vi "PID unit_re.vi"(0 "dt":dbl=1.0 format="%0.2f", 4 "Kd":dbl=30.0, 5 "PID":bool, 6 "현재 온도":dbl[](array[numeric]), 7 "Ki":dbl=50.0, 8 "Kp":dbl=20.0, 9 "Target 온도":dbl=10.0) -> (3 "적정 PRF":dbl=-95.93375)   [LabVIEW 2016]
uses:
  <vilib>/Analysis/2dsp.llb/Derivative x(t).vi
  <vilib>/Analysis/NI_AALPro.lvlib
panel:
  out "Current T":dbl
  out "Integral X":dbl[](array[numeric]) format="%0.2f"
  out "x-y":dbl[](array[numeric])
  out "Sequence(i)":i32
  out "reversed array":dbl[](array[numeric])
  out "Diff":dbl
  out "Temperature chart":dbl(graph)
  out "dX/dt":dbl[](array[numeric]) format="%0.2f"
  out "array w/ subset deleted":dbl[](array[numeric])=[-30.25, -30.5, -30.75, -31.0, -31.25, -31.5, -31.75, -32.0]
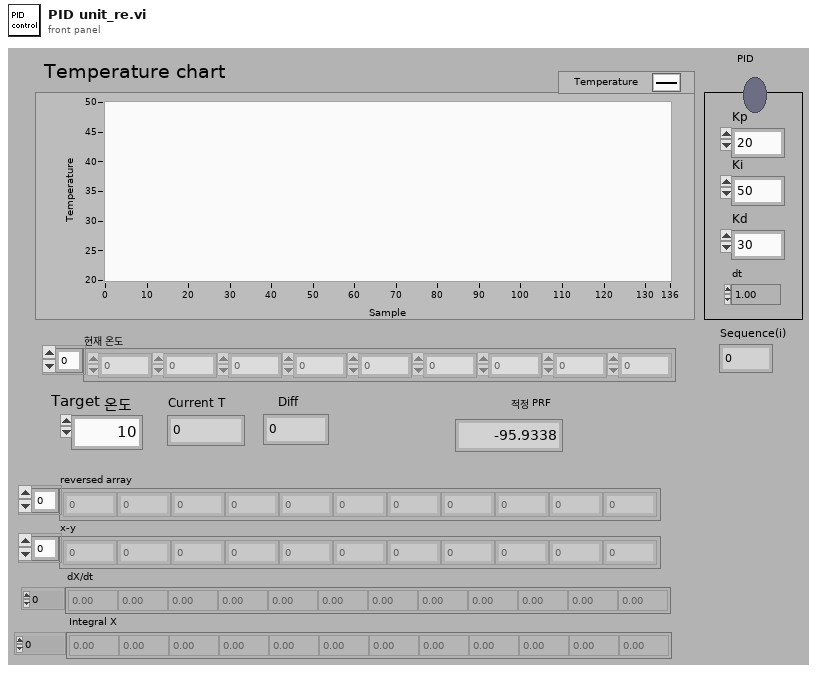
[diagram p1: front panel]
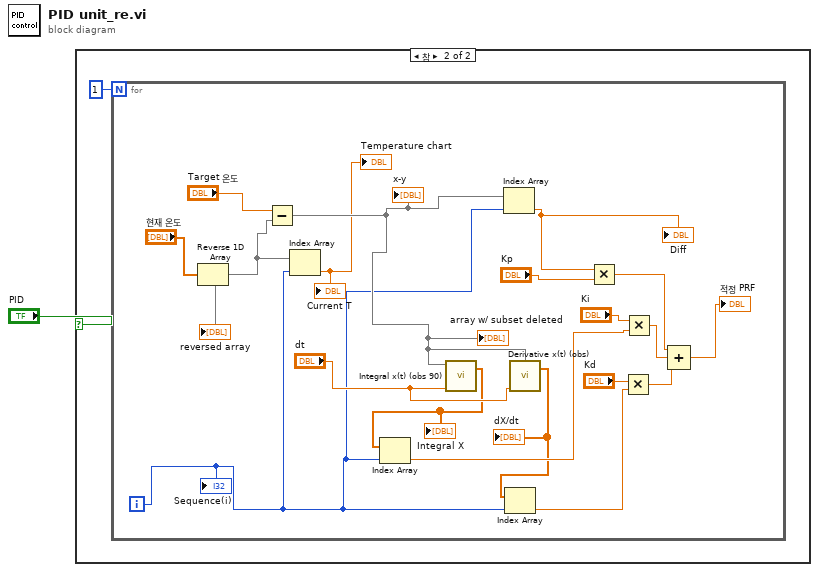
[diagram p0: block diagram]
diagram:
  n1 = case shown="참" "PID" {
    frame False {
    }
    frame True {
      n2 = for {
        N: 1 -> [_]
        i -> [w6]
        n3 = Reverse 1D Array(array="현재 온도") -> (reversed array=w4:dbl[])
        "reversed array" <- w4
        n4 = Subtract(x="Target 온도", y=w4) -> (x-y=w9:dbl[])
        "array w/ subset deleted" <- w9
        "x-y" <- w9
        n5 = Index Array(array=w4, index=w6) -> (element=→"Temperature chart" →"Current T":dbl)
        n6 = call <vilib>:"Integral x(t) (obs 90).vi"("dt"="dt", "X"=w9) -> ("Integral X"=w13:dbl[])  [unwired: 2 in, 1 out]
        "Integral X" <- w13
        n7 = Index Array(array=w13, index=w6) -> (element=w12:dbl)
        n8 = Index Array(array=w9, index=w6) -> (element=w8:dbl)
        "Diff" <- w8
        n9 = call <vilib>:"Derivative x(t) (obs).vi"("dt"="dt", "X"=w9) -> ("dX/dt"=w11:dbl[])  [unwired: 2 in, 1 out]
        "dX/dt" <- w11
        n10 = Index Array(array=w11, index=w6) -> (element=w10:dbl)
        n11 = Multiply(x=w8, y="Kp") -> (x*y=w21:dbl)
        n12 = Multiply(x="Kd", y=w10) -> (x*y=w15:dbl)
        n13 = Multiply(x="Ki", y=w12) -> (x*y=w14:dbl)
        n14 = Compound Arithmetic op=ADD(w21, w14, w15) -> (→"적정 PRF":dbl)
        "Sequence(i)" <- w6
      }
    }
  }
